vi "Get Channel Data.vi"(8 "error in (no error)":errorcluster, 11 "Channel Reference in":u64 format="%.0x") -> (0 "error out":errorcluster, 1 "ChannelSetting":T1={"IOType"=enum."Input", "DefaultValue"=[[0.0]], "Dimensions"={"Row"=1, "Column"=1}, "Units"="", "Description"="", "Faultable"=FALSE}, 2 "Name":string, 3 "Channel Reference out":u64 format="%.0x", 4 "found":bool, 5 "GUID":string, 7 "PathName":string)   [LabVIEW 2013, in "Hierarchy Framework.lvlib" / "Channel.lvclass"]
doc: "Returns information about the channel specified by <B>Channel Reference in</B>."
uses:
  Channel.lvclass
  Ctls/ChannelSetting.ctl
  Ctls/IOType.ctl
  Ctls/Dimensions.ctl
  Generic/Generic.lvclass
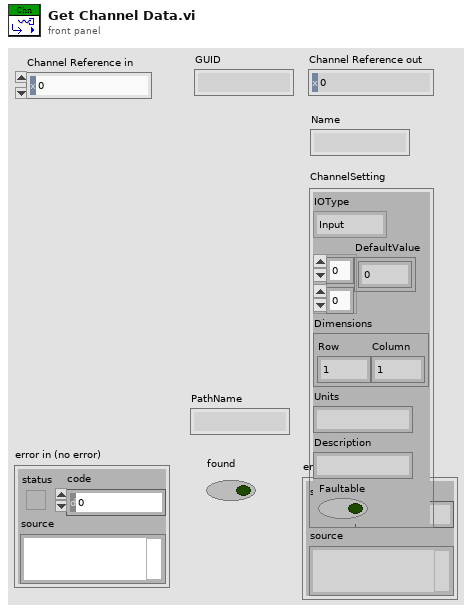
[diagram p1: front panel]
types:
  T1 = typedef "Hierarchy Framework.lvlib/Channel.lvclass/ChannelSetting.ctl" = cluster{"IOType":T2, "DefaultValue":dbl[][], "Dimensions":T3, "Units":string, "Description":string, "Faultable":bool}
  T2 = typedef "Hierarchy Framework.lvlib/Channel.lvclass/IOType.ctl" = enum16{"Input", "Output"}
  T3 = typedef "Hierarchy Framework.lvlib/Channel.lvclass/Dimensions.ctl" = cluster{"Row":i32, "Column":i32}
  T4 = typedef "Framework.lvlib/Channel.lvclass/IOType.ctl" = enum16{"Input", "Output"}
  T5 = typedef "Framework.lvlib/Channel.lvclass/Dimensions.ctl" = cluster{"Row":i32, "Column":i32}
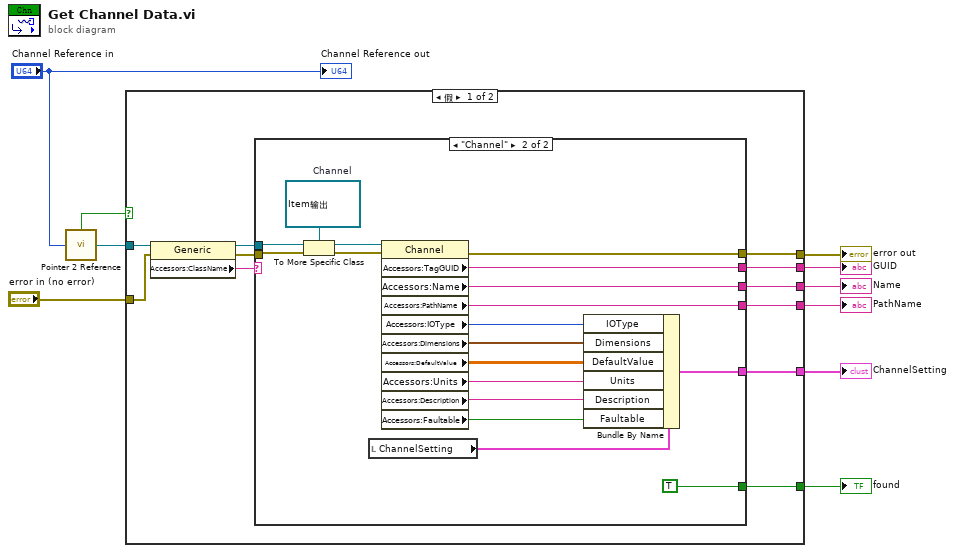
[diagram p0: block diagram]
diagram:
  n1 = call "Pointer 2 Reference.vi"("Pointer"="Channel Reference in") -> ("Not A Refnum?"=w9:bool, "Generic Reference"=w8:refnum<data-value>)
  n2 = case shown="假" w9 {
    tunnel: w8 -> [w21 _]
    tunnel: "error in (no error)" -> [w18 w41]
    tunnel: [w16 _] -> w6
    tunnel: [w15 _] -> w5
    tunnel: [w14 _] -> w4
    tunnel: [w13 _] -> w3
    tunnel: [w12 w41] -> w2
    tunnel: [w11 _] -> w1
    frame False {
      n3 = property class="Generic"(reference=w21, error in=w18) -> (reference out=w19:refnum<data-value>, error out=w17:errorcluster, "Accessors:ClassName"=w20:string)
      n4 = case shown="\"Channel\"" w20 {
        tunnel: w19 -> [_ w40]
        tunnel: w17 -> [w22 w39]
        tunnel: [_ w35] -> w16
        tunnel: [_ w34] -> w15
        tunnel: [_ w33] -> w14
        tunnel: [_ w25] -> w13
        tunnel: [w22 w24] -> w12
        tunnel: [_ TRUE] -> w11
        frame Default {
        }
        frame "Channel" {
          w38 = refnum<data-value> refnum  # Channel
          n5 = To More Specific Class(target class=w38, reference=w40, error in=w39) -> (specific class reference=w37:refnum<data-value>, error out=w36:errorcluster)
          n6 = local read "ChannelSetting"() -> (w32:T1)
          n7 = property class="Channel"(reference=w37, error in=w36) -> (error out=w24:errorcluster, "Accessors:TagGUID"=w35:string, "Accessors:Name"=w34:string, "Accessors:PathName"=w33:string, "Accessors:IOType"=w31:T4, "Accessors:Dimensions"=w30:T5, "Accessors:DefaultValue"=w29:dbl[][], "Accessors:Units"=w28:string, "Accessors:Description"=w27:string, "Accessors:Faultable"=w26:bool)  [unwired: 1 out]
          n8 = Bundle By Name(cluster=w32, "IOType"=w31, "Dimensions"=w30, "DefaultValue"=w29, "Units"=w28, "Description"=w27, "Faultable"=w26) -> (w25:T1)
        }
      }
    }
    frame True {
    }
  }
  "error out" <- w2
  "ChannelSetting" <- w3
  "GUID" <- w6
  "Name" <- w5
  "PathName" <- w4
  "found" <- w1
  "Channel Reference out" <- "Channel Reference in"
